vi "ChannelUI.vi"() -> ()   [LabVIEW 2025, in "Abstract Engine.lvlib" / "Abstract Channel.lvclass"]
doc: "Copyright 2017 National Instruments Corporation\n\nLicensed under the Apache License, Version 2.0 (the \"License\"); you may not use this file except in compliance with the License. You may obtain a copy of the License at http://www.apache.org/licenses/LICENSE-2.0\nUnless required by applicable law or agreed to in writing, software distributed under the License is distributed on an \"AS IS\" BASIS, WITHOUT WARRANTIES OR CONDITIONS OF ANY KIND, either express or implied. See the License for the specific language governing permissions and limitations under the License."
uses:
  Abstract Channel.lvclass
  Users/Public/Documents/Sandia National Labs/TSS Plugin/CEF.lvlibp/Node/NodeRef.ctl
  Users/Public/Documents/Sandia National Labs/TSS Plugin/CEF.lvlibp/Node/CEF_Node.lvclass
  Users/Public/Documents/Sandia National Labs/TSS Plugin/CEF.lvlibp/Node/mainQref.ctl
  Users/Public/Documents/Sandia National Labs/TSS Plugin/CEF.lvlibp/Node/UserEventRef.ctl
  Channel configuration/Default Channel.ctl
  C:/Users/Public/Documents/Sandia National Labs/TSS Plugin/CEF.lvlibp/Node/CEF_Node.lvclass
  Abstract Channel.lvclass/Abstract Channel.ctl
  Channel configuration/Channel configuration.lvclass/Channel configuration.ctl
  Channel configuration/Read Channel Setting.vi
  Channel configuration/Write Channel Setting.vi
  Channel configuration/Channel configuration.lvclass
panel:
  in  "Channel":T1={"Address"="None", "SW Alias"="None", "Description"="* Type = Channel Class", "Enabled"=TRUE, "Type"="None"}
  in  "user event":T2
  in  "main queue":T3
  in  "node ref":T4
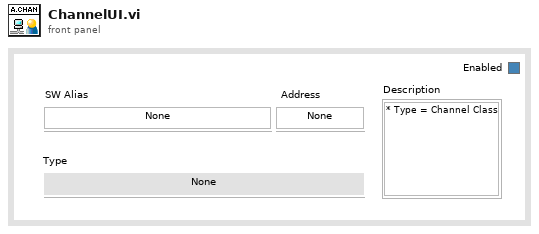
[diagram p1: front panel]
types:
  T1 = typedef "Abstract Engine.lvlib/Channel configuration.lvclass/Default Channel.ctl" = cluster{"Address":string, "SW Alias":string, "Description":string, "Enabled":bool, "Type":string}
  T2 = typedef "CEF.lvlibp/CEF_Node.lvclass/UserEventRef.ctl" = refnum<user-event>
  T3 = typedef "CEF.lvlibp/CEF_Node.lvclass/mainQref.ctl" = refnum<queue>
  T4 = typedef "CEF.lvlibp/CEF_Node.lvclass/NodeRef.ctl" = refnum<data-value>
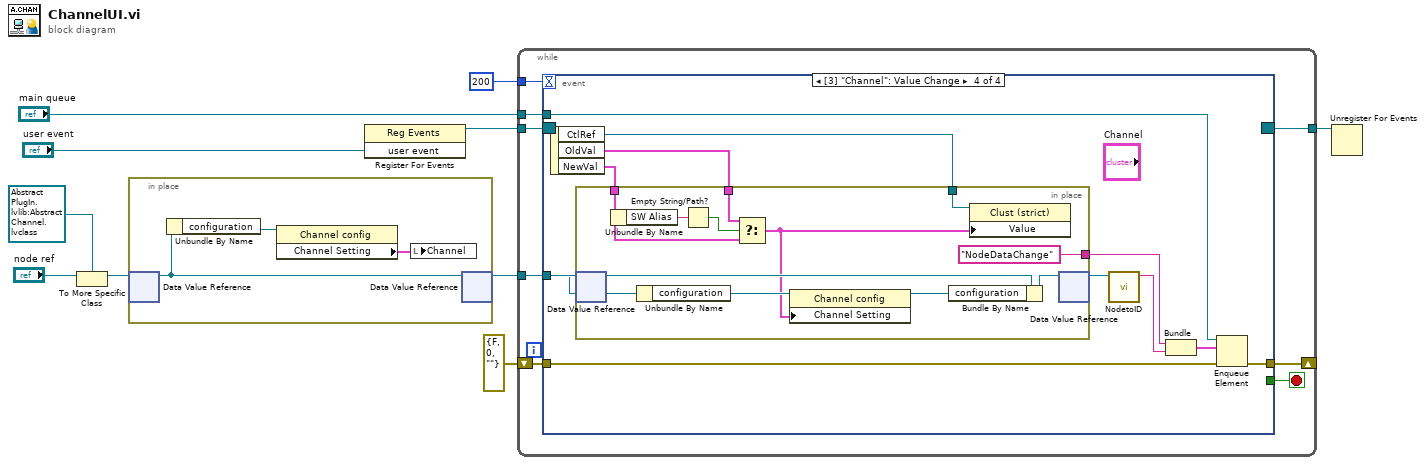
[diagram p0: block diagram]
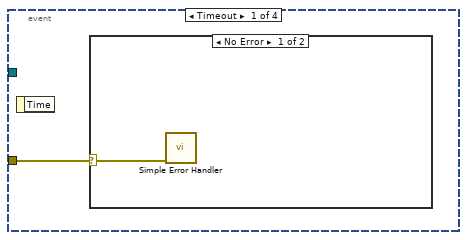
[diagram p2: hidden frame]
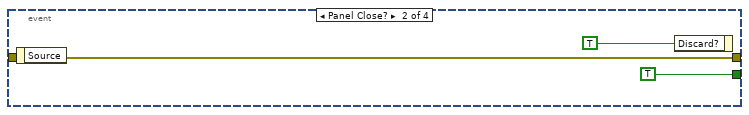
[diagram p4: hidden frame]
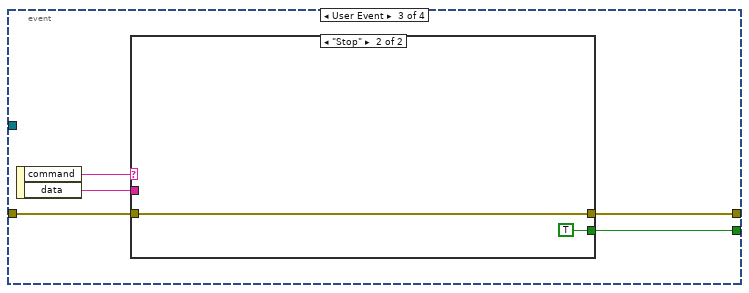
[diagram p5: hidden frame]
diagram:
  n1 = To More Specific Class(target class=refnum<data-value> refnum ("data value reference"), reference="node ref") -> (specific class reference=w6:refnum<data-value>)  [unwired: 1 in, 1 out]
  n2 = in-place {
    # "Initialize the front panel controls when loaded"
    n3 = in-place-dvr #1(w6) -> (w13:refnum<class "Abstract Channel.lvclass">)  [unwired: 1 out]
    n4 = Unbundle By Name(w13) -> ("configuration"=w12:refnum<class "Channel configuration.lvclass">)
    n5 = property class="Channel config"(reference=w12) -> ("Channel Setting"=w11:T1)  [unwired: 1 in, 2 out]
    n6 = local write "Channel"(w11) -> ()
    n7 = in-place-dvr #1(w13) -> (w5:refnum<data-value>)  [unwired: 1 out]
  }
  n8 = register-events("user event") -> (reference out=w9:refnum<event-registration>)  [unwired: 2 in, 1 out]
  n9 = while {
    tunnel: w5 -> [w21]
    tunnel: w9 -> [w20]
    tunnel: [w19] -> w8
    tunnel: "main queue" -> [w15]
    shift-right: [w16] -> _
    shift-left: errorcluster {"status"=FALSE, "code"=0, "source"=""} ("error out") -> [w17]
    tunnel: 200 -> [w14]
    stop <- w18 stop-if-true
    n10 = event shown="[3] \"Channel\": Value Change" {
      selector: w20 -> [_ _ _ _]
      dyn-events: [_ _ _ _] -> w19
      timeout: w14 -> [_ _ _ _]
      tunnel: w21 -> [_ _ _ w43]
      tunnel: [_ TRUE w31 _] -> w18
      tunnel: [_ w24 w27 w44] -> w16
      tunnel: w17 -> [w22 w24 w29 w38]
      tunnel: w15 -> [_ _ _ w45]
      event Timeout {
        n11 = event-data() -> ()  [unwired: 1 in, 1 out]
        n12 = case shown="No Error" w22 {
          selector: w22 -> [w23 _]
          frame No Error {
            n13 = call <vilib>:"Simple Error Handler.vi"("error in (no error)"=w23) -> ()  [unwired: 4 in, 5 out]
          }
          frame Error {
          }
        }
      }
      event Panel Close? {
        n14 = event-data() -> ()  [unwired: 1 in, 1 out]
        n15 = event-data("Discard?"=TRUE) -> ()  [unwired: 1 in, 1 out]
      }
      event User Event {
        n16 = event-data() -> ("command"=w28:string, "data"=w30:string)  [unwired: 1 in]
        n17 = case shown="\"Stop\"" w28 {
          tunnel: [_ TRUE] -> w31
          tunnel: w30 -> [_ _]
          tunnel: w29 -> [w32 w33]
          tunnel: [w32 w33] -> w27
          frame Default {
          }
          frame "Stop" {
          }
        }
      }
      event Value Change {
        n18 = event-data() -> ("CtlRef"=w39:refnum<vi>, "OldVal"=w40:T1, "NewVal"=w41:T1)  [unwired: 1 in]
        n19 = in-place {
          in-place-border: w41 -> [w50]
          in-place-border: w40 -> [w49]
          in-place-border: w39 -> [w48]
          in-place-border: ["NodeDataChange" ("Message Name")] -> w37
          n20 = in-place-dvr #2(w43) -> (w56:refnum<class "Abstract Channel.lvclass">)  [unwired: 1 out]
          n21 = Unbundle By Name(w50) -> ("SW Alias"=w52:string)
          n22 = Unbundle By Name(w56) -> ("configuration"=w55:refnum<class "Channel configuration.lvclass">)
          n23 = Empty String/Path?(string/path=w52) -> (empty?=w51:bool)
          n24 = Select(t=w49, s=w51, f=w50) -> (s? t:f=w47:T1)
          n25 = property class="Channel config"(reference=w55, "Channel Setting"=w47) -> (reference out=w53:refnum<class "Channel configuration.lvclass">)  [unwired: 1 in, 1 out]
          n26 = Bundle By Name(cluster=w56, "configuration"=w53) -> (w54:refnum<class "Abstract Channel.lvclass">)
          n27 = property class="Clust (strict)"(reference=w48, "Value"=w47) -> ()  [unwired: 1 in, 2 out]
          n28 = in-place-dvr #2(w54) -> (w42:refnum<data-value>)  [unwired: 1 out]
        }
        n29 = call "NodetoID.vi"("node ref"=w42) -> ("ID"=w36:string)  [unwired: 9 in, 1 out]
        n30 = Bundle("Message Name"=w37, "ID"=w36) -> (w35:cluster{"Message Name":string, "ID":string})  [unwired: 1 in]
        n31 = Enqueue Element(queue=w45, element=w35, error in (no error)=w38) -> (error out=w44:errorcluster)  [unwired: 1 in, 2 out]
      }
    }
  }
  n32 = Unregister For Events(event registration refnum=w8) -> ()  [unwired: 1 in, 1 out]
